vi "Burst_manual.vi"() -> ()   [LabVIEW 2019, in "Prueba08.lvclass"]
uses:
  Prueba08.lvclass
  ClusterGEN.ctl
  Instrumento/DS360/DS360.lvclass
panel:
  out "# ciclos":i32
  out "error out":errorcluster
  in  "error in (no error)":errorcluster
  in  "input cluster":T1
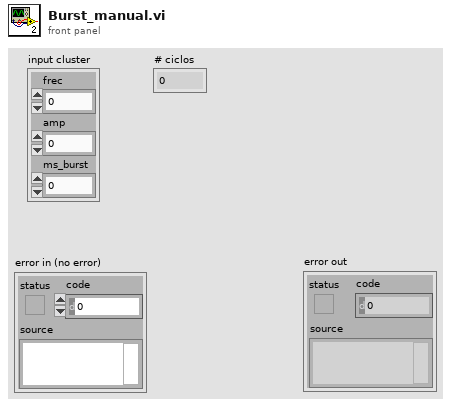
[diagram p1: front panel]
types:
  T1 = typedef "Prueba08.lvclass/ClusterGEN.ctl" = cluster{"frec":dbl, "amp":dbl, "ms_burst":dbl}
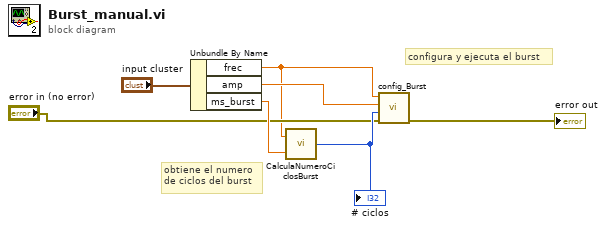
[diagram p0: block diagram]
diagram:
  # "configura y ejecuta el burst"
  # "obtiene el numero\nde ciclos del burst"
  n1 = Unbundle By Name("input cluster") -> ("frec"=w1:dbl, "amp"=w6:dbl, "ms_burst"=w7:dbl)
  n2 = call "CalculaNumeroCiclosBurst.vi"("ms_burst"=w7, "frec"=w1) -> ("# ciclos"=w5:i32)
  "# ciclos" <- w5
  n3 = call "config_Burst.vi"("error in (no error)"="error in (no error)", "# ciclos"=w5, "Amplitud (Vrms)"=w6, "Frec (Hz)"=w1) -> ("error out"=→"error out":errorcluster)  [unwired: 6 in, 1 out]
